vi "Get Marker State.vi"(8 "Error In":errorcluster) -> (0 "Error Out":errorcluster, 3 "Marker State Out":T1)   [LabVIEW 2014]
uses:
  Controls/GMap Marker State.ctl
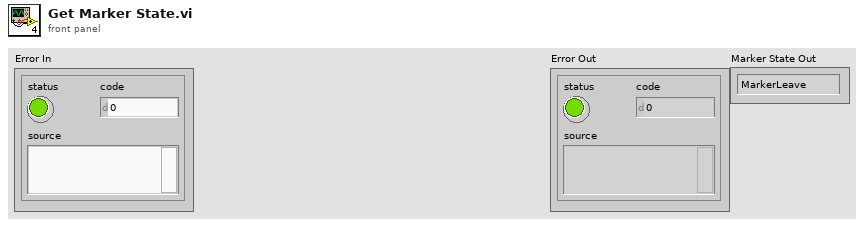
[diagram p1: front panel]
types:
  T1 = typedef "GMap Marker State.ctl" = enum16{"MarkerLeave", "MarkerEntered"}
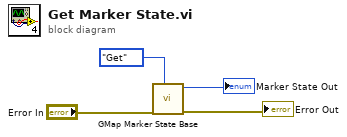
[diagram p0: block diagram]
diagram:
  n1 = call "GMap Marker State Base.vi"("Method"=enum16{"Get", "Set"}."Get", "Error In"="Error In") -> ("Error Out"=→"Error Out":errorcluster, "Marker State Out"=→"Marker State Out":T1)  [unwired: 8 in]
